vi "condition3dplot_v02.vi"(8 "error in":errorcluster, 11 "3d graph":refnum<k7>) -> (0 "error out":errorcluster, 3 "3d graph out":refnum<k7>)   [LabVIEW 2015]
uses:
  <vilib>/Platform/NI_3dgraph.lvlib
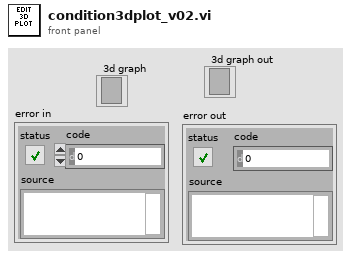
[diagram p1: front panel]
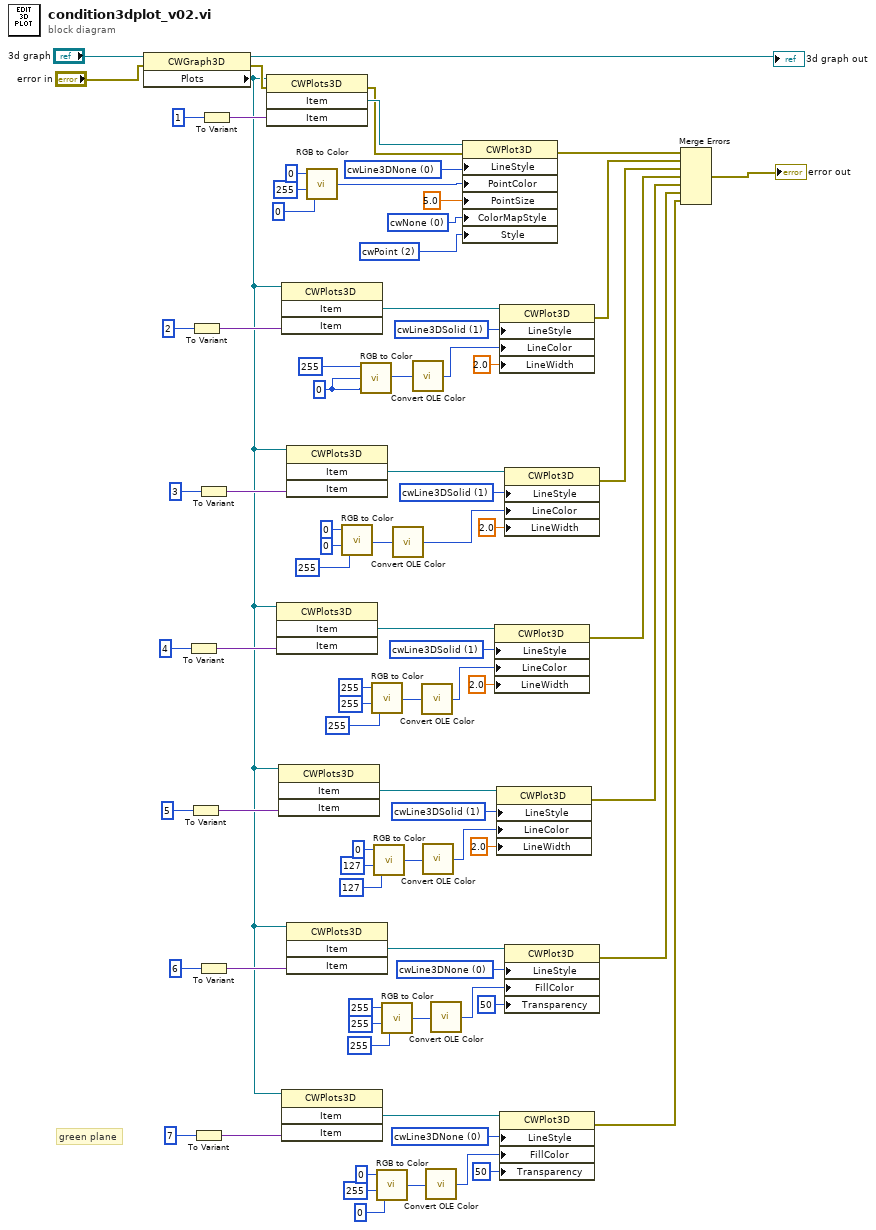
[diagram p0: block diagram]
diagram:
  w7 = 0 items=["cwLine3DNone"=0, "cwLine3DSolid"=1, "cwLine3DDash"=4, "cwLine3DDot"=5, "cwLine3DDashDot"=6] ("LineStyle")
  w17 = 0 items=["cwLine3DNone"=0, "cwLine3DSolid"=1, "cwLine3DDash"=4, "cwLine3DDot"=5, "cwLine3DDashDot"=6] ("LineStyle")
  w28 = u8 0 ("B")
  w44 = 1 items=["cwLine3DNone"=0, "cwLine3DSolid"=1, "cwLine3DDash"=4, "cwLine3DDot"=5, "cwLine3DDashDot"=6] ("LineStyle")
  w49 = 1 items=["cwLine3DNone"=0, "cwLine3DSolid"=1, "cwLine3DDash"=4, "cwLine3DDot"=5, "cwLine3DDashDot"=6] ("LineStyle")
  w62 = 1 items=["cwLine3DNone"=0, "cwLine3DSolid"=1, "cwLine3DDash"=4, "cwLine3DDot"=5, "cwLine3DDashDot"=6] ("LineStyle")
  w65 = 1 items=["cwLine3DNone"=0, "cwLine3DSolid"=1, "cwLine3DDash"=4, "cwLine3DDot"=5, "cwLine3DDashDot"=6] ("LineStyle")
  w76 = 2 items=["cwLine"=1, "cwPoint"=2, "cwLinePoint"=3, "cwHiddenLine"=4, "cwSurface"=5, "cwSurfaceLine"=6, "cwSurfaceNormal"=7, "cwContourLine"=8, "cwSurfaceContour"=9] ("Style")
  w77 = 0 items=["cwNone", "cwShaded", "cwColorSpectrum", "cwGrayScale", "cwCustom"] ("ColorMapStyle")
  w81 = 0 items=["cwLine3DNone"=0, "cwLine3DSolid"=1, "cwLine3DDash"=4, "cwLine3DDot"=5, "cwLine3DDashDot"=6] ("LineStyle")
  # "green plane"
  n1 = property class="CWGraph3D"(reference="3d graph", error in="error in") -> (reference out=→"3d graph out":refnum<k7>, error out=w75:errorcluster, "Plots"=w12:refnum<k7>)
  n2 = To Variant(anything=4) -> (Variant=w54:variant)
  n3 = To Variant(anything=5) -> (Variant=w39:variant)
  n4 = To Variant(anything=2) -> (Variant=w67:variant)
  n5 = To Variant(anything=7) -> (Variant=w2:variant)
  n6 = To Variant(anything=3) -> (Variant=w57:variant)
  n7 = To Variant(anything=6) -> (Variant=w22:variant)
  n8 = To Variant(anything=1) -> (Variant=w83:variant)
  n9 = invoke class="CWPlots3D" method="Item"(reference=w12, error in=w75, "Item"=w83) -> (error out=w74:errorcluster, "Item"=w82:refnum<k7>)  [unwired: 1 in, 2 out]
  n10 = invoke class="CWPlots3D" method="Item"(reference=w12, "Item"=w54) -> ("Item"=w53:refnum<k7>)  [unwired: 2 in, 3 out]
  n11 = invoke class="CWPlots3D" method="Item"(reference=w12, "Item"=w39) -> ("Item"=w40:refnum<k7>)  [unwired: 2 in, 3 out]
  n12 = invoke class="CWPlots3D" method="Item"(reference=w12, "Item"=w67) -> ("Item"=w66:refnum<k7>)  [unwired: 2 in, 3 out]
  n13 = invoke class="CWPlots3D" method="Item"(reference=w12, "Item"=w2) -> ("Item"=w3:refnum<k7>)  [unwired: 2 in, 3 out]
  n14 = invoke class="CWPlots3D" method="Item"(reference=w12, "Item"=w57) -> ("Item"=w58:refnum<k7>)  [unwired: 2 in, 3 out]
  n15 = invoke class="CWPlots3D" method="Item"(reference=w12, "Item"=w22) -> ("Item"=w21:refnum<k7>)  [unwired: 2 in, 3 out]
  n16 = call <vilib>:"RGB to Color.vi"("B"=u8 0, "G"=u8 255, "R"=u8 0) -> ("Color"=w69:u32)
  n17 = call <vilib>:"RGB to Color.vi"("B"=u8 255, "G"=u8 0, "R"=u8 0) -> ("Color"=w27:u32)
  n18 = call <vilib>:"RGB to Color.vi"("B"=w28, "G"=w28, "R"=u8 255 ("G")) -> ("Color"=w31:u32)
  n19 = call <vilib>:"RGB to Color.vi"("B"=u8 255, "G"=u8 255, "R"=u8 255) -> ("Color"=w25:u32)
  n20 = call <vilib>:"RGB to Color.vi"("B"=u8 127, "G"=u8 127, "R"=u8 0) -> ("Color"=w45:u32)
  n21 = call <vilib>:"RGB to Color.vi"("B"=u8 0, "G"=u8 255, "R"=u8 0) -> ("Color"=w8:u32)
  n22 = call <vilib>:"RGB to Color.vi"("B"=u8 255, "G"=u8 255, "R"=u8 255) -> ("Color"=w16:u32)
  n23 = call <vilib>:"Convert OLE Color.vi"("color in"=w27) -> ("color out"=w26:u32)
  n24 = call <vilib>:"Convert OLE Color.vi"("color in"=w31) -> ("color out"=w30:u32)
  n25 = call <vilib>:"Convert OLE Color.vi"("color in"=w25) -> ("color out"=w24:u32)
  n26 = call <vilib>:"Convert OLE Color.vi"("color in"=w45) -> ("color out"=w46:u32)
  n27 = call <vilib>:"Convert OLE Color.vi"("color in"=w8) -> ("color out"=w9:u32)
  n28 = call <vilib>:"Convert OLE Color.vi"("color in"=w16) -> ("color out"=w15:u32)
  n29 = property class="CWPlot3D"(reference=w82, error in=w74, "LineStyle"=w81, "PointColor"=w69, "PointSize"=5.0, "ColorMapStyle"=w77, "Style"=w76) -> (error out=w37:errorcluster)  [unwired: 1 out]
  n30 = property class="CWPlot3D"(reference=w53, "LineStyle"=w49, "LineColor"=w24, "LineWidth"=2.0) -> (error out=w34:errorcluster)  [unwired: 1 in, 1 out]
  n31 = property class="CWPlot3D"(reference=w40, "LineStyle"=w44, "LineColor"=w46, "LineWidth"=2.0) -> (error out=w33:errorcluster)  [unwired: 1 in, 1 out]
  n32 = property class="CWPlot3D"(reference=w66, "LineStyle"=w65, "LineColor"=w30, "LineWidth"=2.0) -> (error out=w36:errorcluster)  [unwired: 1 in, 1 out]
  n33 = property class="CWPlot3D"(reference=w3, "LineStyle"=w7, "FillColor"=w9, "Transparency"=50) -> (error out=w11:errorcluster)  [unwired: 1 in, 1 out]
  n34 = property class="CWPlot3D"(reference=w58, "LineStyle"=w62, "LineColor"=w26, "LineWidth"=2.0) -> (error out=w35:errorcluster)  [unwired: 1 in, 1 out]
  n35 = property class="CWPlot3D"(reference=w21, "LineStyle"=w17, "FillColor"=w15, "Transparency"=50) -> (error out=w14:errorcluster)  [unwired: 1 in, 1 out]
  n36 = Merge Errors(w37, w36, w35, w34, w33, w14, w11) -> (→"error out":errorcluster)
